vi "ni579x Read EEPROM Calibration Header.vi"(0 "Register Bus":T2, 1 "scope":string(combo)="characterization data eeprom", 5 "start address":u32 format="%x", 11 "Error In":errorcluster) -> (4 "Register Bus (out)":T2, 6 "EEPROM Calibration Header":T1={"Checksum"=0, "Date"=timestamp(0 s since 1904-01-01), "Temperature"=0.0, "Misc. Info"="", "Pointer to Device Data Header"=0, "Number of Reserved Bytes"=28} {"Checksum" format="%x"}, 15 "Error Out":errorcluster)   [LabVIEW 2015, in "ni579x Config v2 Host.lvlib"]
uses:
  <instrlib>/ni579x/Config/v2/Host/ni579x Config v2 Host.lvlib
  <instrlib>/_niInstr/Register Bus/v0/Host/Public/Register Bus Session.ctl
  <instrlib>/_niInstr/Register Bus/v0/Host/Private/Session Data.ctl
  <instrlib>/ni579x/Config/v2/Shared/Types/EEPROM/ni579x EEPROM Calibration Header.ctl
  <instrlib>/ni579x/Config/v2/Shared/Conversions/From Byte Array (U32).vi
  <instrlib>/ni579x/Config/v2/Shared/Conversions/From Byte Array (F32).vi
  <instrlib>/ni579x/Config/v2/Shared/Conversions/From Byte Array (LV Timestamp).vi
  <instrlib>/ni579x/Config/v2/Shared/ni579x Config v2 Shared.lvlib
  <instrlib>/_niInstr/Register Bus/v0/Host/niInstr Register Bus v0 Host.lvlib
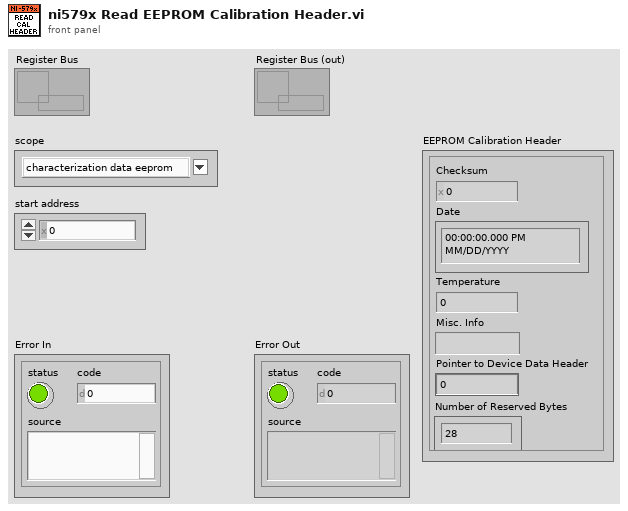
[diagram p1: front panel]
types:
  T1 = typedef "ni579x Config v2 Shared.lvlib/ni579x EEPROM Calibration Header.ctl" = cluster{"Checksum":u32, "Date":timestamp, "Temperature":sgl, "Misc. Info":string, "Pointer to Device Data Header":u32, "Number of Reserved Bytes":i32}
  T2 = typedef "niInstr Register Bus v0 Host.lvlib/Register Bus Session.ctl" = refnum<queue>
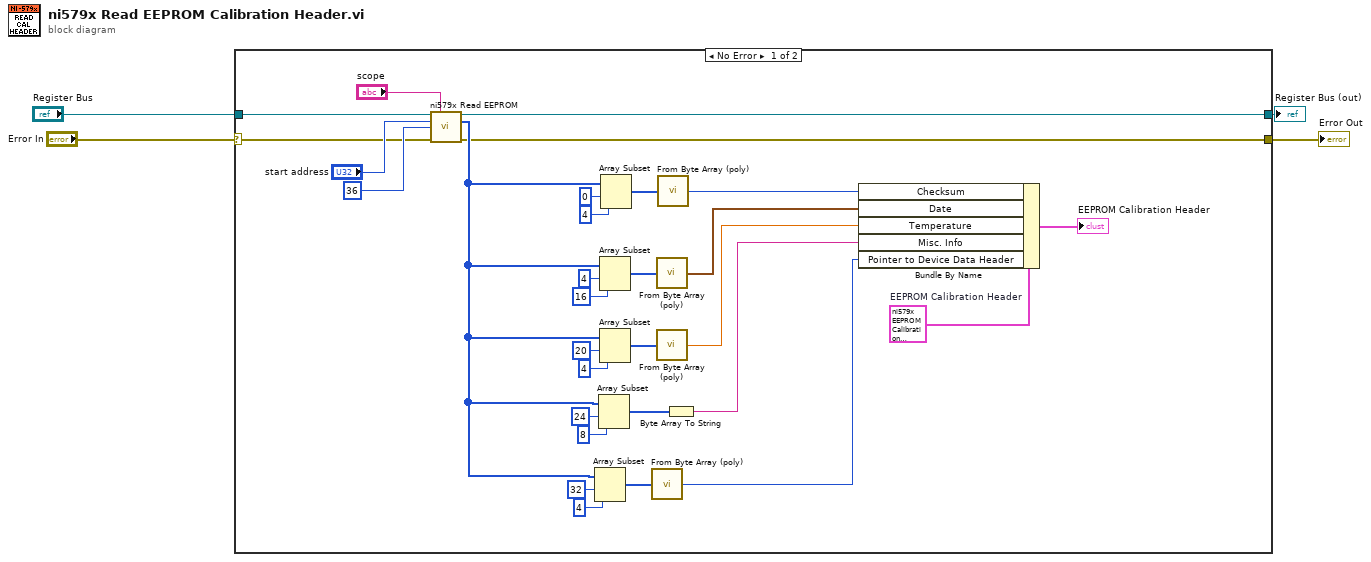
[diagram p0: block diagram]
diagram:
  n1 = case shown="No Error" "Error In" {
    selector: "Error In" -> [w31 w36]
    tunnel: [w11 w36] -> w3
    tunnel: "Register Bus" -> [w32 w35]
    tunnel: [w12 w35] -> w1
    frame No Error {
      w9 = T1 {"Checksum"=0, "Date"=timestamp(0 s since 1904-01-01), "Temperature"=0.0, "Misc. Info"="", "Pointer to Device Data Header"=0, "Number of Reserved Bytes"=28}  # EEPROM Calibration Header
      n2 = call <instrlib>:"ni579x Read EEPROM.vi"("Register Bus"=w32, "scope"="scope", "start address"="start address", "size"=u32 36, "Error In"=w31) -> ("Register Bus (out)"=w12:T2, "data"=w13:u8[], "Error Out"=w11:errorcluster)  [unwired: 8 in]
      n3 = Array Subset(array=w13, index=32, length=4) -> (w14:u8[])
      n4 = Array Subset(array=w13, index=24, length=8) -> (w17:u8[])
      n5 = Array Subset(array=w13, index=4, length=16) -> (w26:u8[])
      n6 = Array Subset(array=w13, index=20, length=4) -> (w21:u8[])
      n7 = Array Subset(array=w13, index=0, length=4) -> (w28:u8[])
      n8 = call-poly <instrlib>:"From Byte Array (poly).vi"("byte array in"=w14) -> ("element out"=w6:u32)
      n9 = call-poly <instrlib>:"From Byte Array (poly).vi"("byte array in"=w26) -> ("element out"=w20:timestamp)
      n10 = call-poly <instrlib>:"From Byte Array (poly).vi"("byte array in"=w21) -> ("element out"=w8:sgl)
      n11 = call-poly <instrlib>:"From Byte Array (poly).vi"("byte array in"=w28) -> ("element out"=w27:u32)
      n12 = Byte Array To String(unsigned byte array=w17) -> (string=w7:string)
      n13 = Bundle By Name(cluster=w9, "Checksum"=w27, "Date"=w20, "Temperature"=w8, "Misc. Info"=w7, "Pointer to Device Data Header"=w6) -> (→"EEPROM Calibration Header":T1)
    }
    frame Error {
    }
  }
  "Register Bus (out)" <- w1
  "Error Out" <- w3
